vi "LogEngine.vi"(7 "dir path to file":path, 9 "Log Enum":T1=enum."Init", 10 "LogDataIN":string, 11 "cumul time":u32) -> ()   [LabVIEW 8.6]
uses:
  EnumLog.ctl
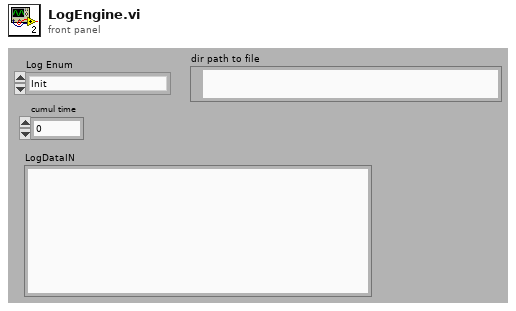
[diagram p1: front panel]
types:
  T1 = typedef "EnumLog.ctl" = enum16{"Idle", "Log", "Init", "AddWP", "Stop", "CleanUp"}
  T2 = enum16{"open", "replace", "create", "open or create", "replace or create", "replace or create with confirmation"}
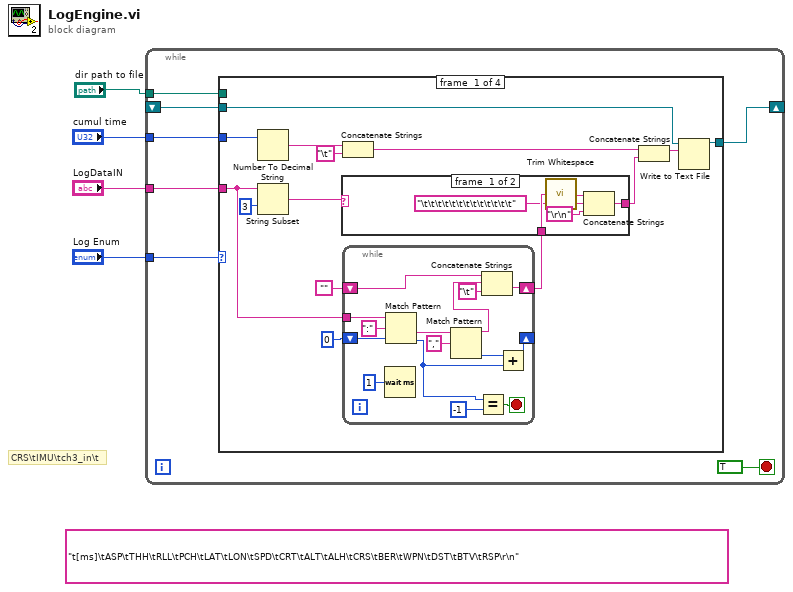
[diagram p0: block diagram]
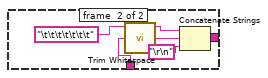
[diagram p2: hidden frame]
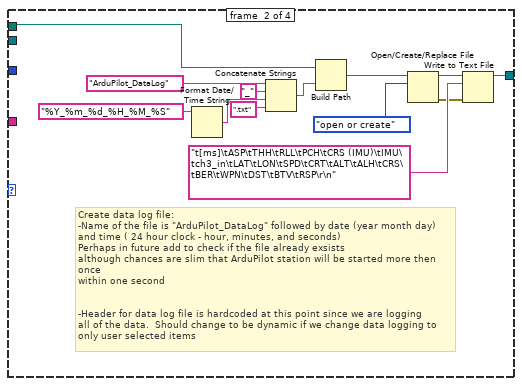
[diagram p3: hidden frame]
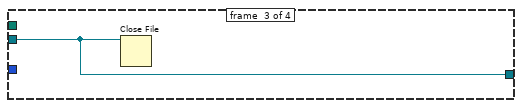
[diagram p4: hidden frame]
diagram:
  (unwired) "t[ms]\tASP\tTHH\tRLL\tPCH\tLAT\tLON\tSPD\tCRT\tALT\tALH\tCRS\tBER\tWPN\tDST\tBTV\tRSP\r\n" ("name (unnamed)")
  # "CRS\\tIMU\\tch3_in\\t"
  n1 = while {
    tunnel: "Log Enum" -> [w10]
    shift-right: [w9] -> _
    shift-left: _ -> [w8]
    tunnel: "cumul time" -> [w7]
    tunnel: "LogDataIN" -> [w6]
    tunnel: "dir path to file" -> [w5]
    stop <- TRUE ("stop") stop-if-true
    n2 = case shown="\"Init\"" w10 {
      tunnel: [w13 w57 w64 w65] -> w9
      tunnel: w8 -> [w12 _ w64 w65]
      tunnel: w7 -> [w15 _ _ _]
      tunnel: w6 -> [w14 _ _ _]
      tunnel: w5 -> [_ w51 _ _]
      frame #0 {
        n3 = Number To Decimal String(number=w15) -> (decimal integer string=w20:string)  [unwired: 1 in]
        n4 = String Subset(string=w14, length (rest)=3 ("length (rest)")) -> (substring=w22:string)  [unwired: 1 in]
        n5 = Concatenate Strings(w20, "\t" ("string")) -> (w17:string)
        n6 = while {
          tunnel: w14 -> [w50]
          shift-right: [w37] -> _
          shift-left: 0 ("offset (0)") -> [w46]
          shift-right: [w45] -> w21
          shift-left: "" -> [w42]
          stop <- w41 stop-if-true
          n7 = Wait (ms)(milliseconds to wait=u32 1) -> ()  [unwired: 1 out]
          n8 = Match Pattern(string=w50, regular expression=":", offset (0)=w46) -> (after substring=w47:string, offset past match=w38:i32)  [unwired: 2 out]
          n9 = Match Pattern(string=w47, regular expression=",") -> (before substring=w44:string, offset past match=w39:i32)  [unwired: 1 in, 2 out]
          n10 = Equal?(x=w38, y=-1) -> (x = y?=w41:bool)
          n11 = Concatenate Strings(w42, w44, "\t" ("string")) -> (w45:string)
          n12 = Add(x=w39, y=w38) -> (x+y=w37:i32)
        }
        n13 = case shown="\"!!!\"" w22 {
          tunnel: [w29 w31] -> w18
          tunnel: w21 -> [w28 w33]
          frame #0 {
            n14 = call <vilib>:"Trim Whitespace.vi"("string"=w28) -> ("trimmed string"=w27:string)  [unwired: 1 in]
            n15 = Concatenate Strings(w27, "\t\t\t\t\t\t\t\t\t\t\t\t\t" ("name"), "\r\n") -> (w29:string)
          }
          frame #1 {
            n16 = call <vilib>:"Trim Whitespace.vi"("string"=w33) -> ("trimmed string"=w35:string)  [unwired: 1 in]
            n17 = Concatenate Strings("\t\t\t\t\t\t\t" ("name"), w35, "\r\n") -> (w31:string)
          }
        }
        n18 = Concatenate Strings(w17, w18) -> (w16:string)
        n19 = Write to Text File(file (use dialog)=w12, text=w16) -> (refnum out=w13:refnum<file>)  [unwired: 2 in, 2 out]
      }
      frame #1 {
        # "Create data log file:\n-Name of the file is \"ArduPilot_DataLog\" followed by date (year month day) \nand time ( 24 hour clock - hour, minutes, and seconds)\nPerhaps in future add to check if the file already exsists\nalthough chances are slim that ArduPilot station will be started more then once\nwithin one second\n\n\n-Header for data log file is hardcoded at this point since we are logging\nall of the data.  Should change to be dynamic if we change data logging to \nonly user selected items"
        n20 = Format Date/Time String(time format string (%c)="%Y_%m_%d_%H_%M_%S") -> (date/time string=w53:string)  [unwired: 2 in]
        n21 = Concatenate Strings("ArduPilot_DataLog" ("name or relative path"), "_" ("string"), w53, ".txt" ("string")) -> (w55:string)
        n22 = Build Path(base path=w51, name or relative path=w55) -> (appended path=w61:path)
        n23 = Open/Create/Replace File(file path (use dialog)=w61, operation (0:open)=T2."open or create") -> (refnum out=w59:refnum<file>, error out=w58:errorcluster)  [unwired: 4 in, 1 out]
        n24 = Write to Text File(file (use dialog)=w59, text="t[ms]\tASP\tTHH\tRLL\tPCH\tCRS (IMU)\tIMU\tch3_in\tLAT\tLON\tSPD\tCRT\tALT\tALH\tCRS\tBER\tWPN\tDST\tBTV\tRSP\r\n" ("name (unnamed)"), error in=w58) -> (refnum out=w57:refnum<file>)  [unwired: 1 in, 2 out]
      }
      frame #2 {
        n25 = Close File(refnum=w64) -> ()  [unwired: 1 in, 2 out]
      }
      frame #3 {
      }
    }
  }
